vi "Add New Menu Item.vi"(0 "Base Path":path, 7 "Old Value":u16, 11 "Ring Menu Ref":refnum<vi>, 13 "Label or Caption":string) -> (4 "Menu Strings":string[](array[string]), 8 "New Item":string, 10 "Menu Value":u16, 15 "Error Out":errorcluster)   [LabVIEW 2016]
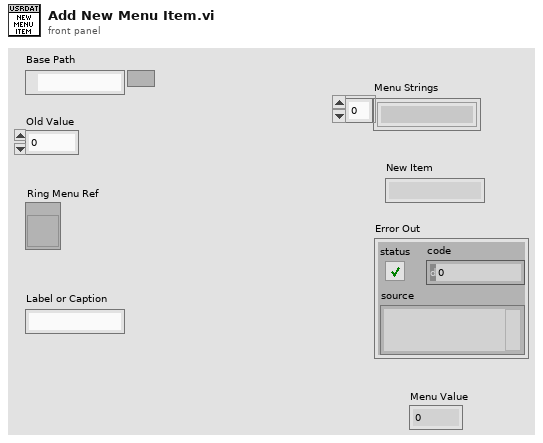
[diagram p1: front panel]
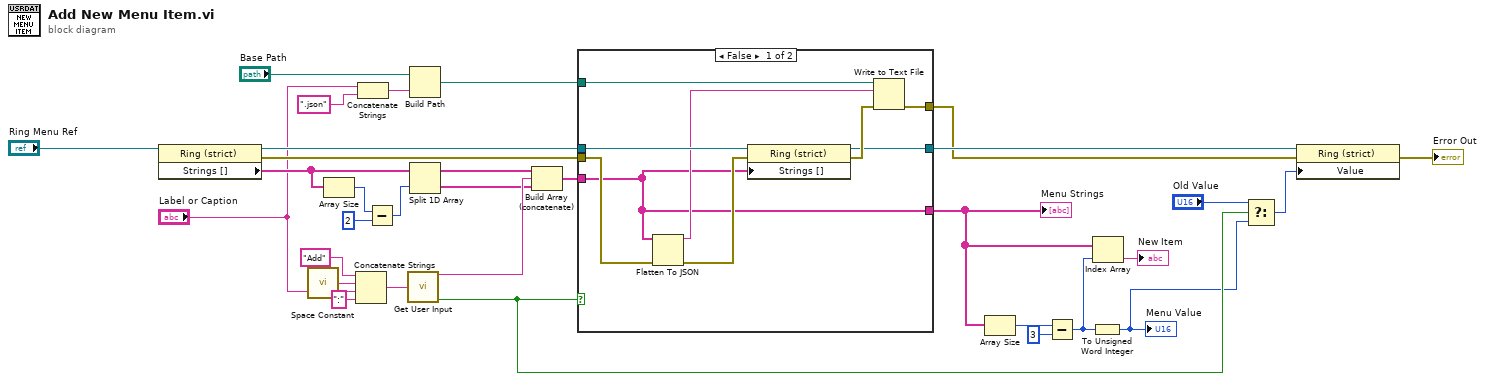
[diagram p0: block diagram]
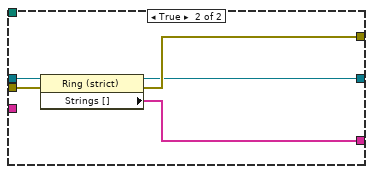
[diagram p2: hidden frame]
diagram:
  n1 = property class="Ring (strict)"(reference="Ring Menu Ref") -> (reference out=w20:refnum<vi>, error out=w18:errorcluster, "Strings []"=w19:string[])  [unwired: 1 in]
  n2 = call <vilib>:"Space Constant.vi"() -> ("String"=w31:string)
  n3 = Array Size(array=w19) -> (size(s)=w10:i32)
  n4 = Concatenate Strings("Add" ("string"), w31, "Label or Caption", ":" ("string")) -> (w29:string)
  n5 = Concatenate Strings("Label or Caption", ".json") -> (w24:string)
  n6 = Subtract(x=w10, y=2) -> (x-y=w11:i32)
  n7 = call "Get User Input.vi"("Dialog Message"=w29) -> ("User Input"=w27:string, "Canceled?"=w6:bool)  [unwired: 13 in]
  n8 = Build Path(base path="Base Path", name or relative path=w24) -> (appended path=w23:path)
  n9 = Split 1D Array(array=w19, index=w11) -> (first subarray=w28:string[], second subarray=w8:string[])
  n10 = Build Array (concatenate)(w28, w27, w8) -> (w25:string[])
  n11 = case shown="False" w6 {
    tunnel: w20 -> [w41 w46]
    tunnel: w25 -> [w34 _]
    tunnel: w23 -> [w40 _]
    tunnel: [w36 w45] -> w2
    tunnel: w18 -> [w35 w44]
    tunnel: [w34 w43] -> w14
    tunnel: [w33 w42] -> w7
    frame False {
      n12 = Flatten To JSON(anything=w34, error in (no error)=w35) -> (JSON string=w37:string, 11:w39:errorcluster)  [unwired: 1 in]
      n13 = property class="Ring (strict)"(reference=w41, error in=w39, "Strings []"=w34) -> (reference out=w33:refnum<vi>, error out=w38:errorcluster)
      n14 = Write to Text File(file (use dialog)=w40, text=w37, error in=w38) -> (error out=w36:errorcluster)  [unwired: 1 in, 2 out]
    }
    frame True {
      n15 = property class="Ring (strict)"(reference=w46, error in=w44) -> (reference out=w42:refnum<vi>, error out=w45:errorcluster, "Strings []"=w43:string[])
    }
  }
  "Menu Strings" <- w14
  n16 = Array Size(array=w14) -> (size(s)=w16:i32)
  n17 = Subtract(x=w16, y=3) -> (x-y=w13:i32)
  n18 = To Unsigned Word Integer(number=w13) -> (unsigned 16bit integer=w4:u16)
  "Menu Value" <- w4
  n19 = Index Array(array=w14, index=w13) -> (element=→"New Item":string)
  n20 = Select(t="Old Value", s=w6, f=w4) -> (s? t:f=w3:u16)
  n21 = property class="Ring (strict)"(reference=w7, error in=w2, "Value"=w3) -> (error out=→"Error Out":errorcluster)  [unwired: 1 out]
